vi "get_FTPSettings_p.vi"(0 "MoAgSy_Host":refnum<class "MoAgSy_Host.lvclass">, 5 "error in (no error)":errorcluster) -> (14 "dup MoAgSy_Host":refnum<class "MoAgSy_Host.lvclass">, 16 "FTP Settings":T1, 19 "error out":errorcluster)   [LabVIEW 2009, in "MoAgSy.lvlib" / "MoAgSy_Host.lvclass"]
doc: "<B>protected</B> VI returns FTP settings of mobile host class.\nIs called by public get ftp settings VI\n\nF.Berck@gsi.de\nGSI Darmstadt 2009"
uses:
  MoAgSy_Host.lvclass
  MoAgSy_Host.lvclass/MoAgSy_Host.ctl
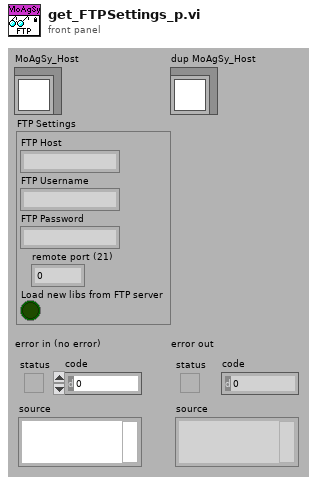
[diagram p1: front panel]
types:
  T1 = cluster{"FTP Host":string, "FTP Username":string, "FTP Password":string, "remote port (21)":u16, "Load new libs from FTP server":bool}
  T2 = cluster{"FTP Host":string, "FTP Username":string, "FTP Password":string, "remote port (21)":u16, "Load new libs from FTP Server":bool}
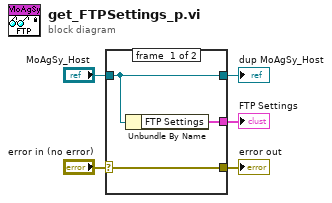
[diagram p0: block diagram]
diagram:
  n1 = case shown="No Error" "error in (no error)" {
    selector: "error in (no error)" -> [w8 w9]
    tunnel: [w8 w9] -> w4
    tunnel: [w7 w10] -> w2
    tunnel: "MoAgSy_Host" -> [w7 w10]
    tunnel: [w6 _] -> w1
    frame #0 {
      n2 = Unbundle By Name(w7) -> ("FTP Settings"=w6:T2)
    }
    frame #1 {
    }
  }
  "error out" <- w4
  "dup MoAgSy_Host" <- w2
  "FTP Settings" <- w1
